vi "ramped_pulse.vi"(8 "error in":errorcluster, 10 "d ramp":u16=1, 11 "d stim":u16=1000) -> (0 "error out":errorcluster, 3 "output":dbl[](array[numeric]))   [LabVIEW 2016]
uses:
  <vilib>/Analysis/1siggen.llb/Ramp Pattern by Samples.vi
  <vilib>/Analysis/NI_AALBase.lvlib
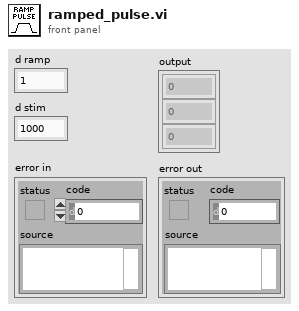
[diagram p1: front panel]
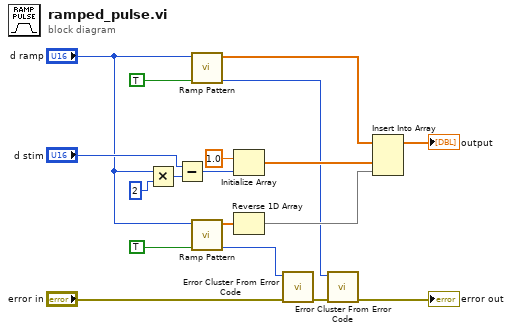
[diagram p0: block diagram]
diagram:
  n1 = Multiply(x="d ramp", y=2 ("d ramp")) -> (x*y=w9:i32)
  n2 = Subtract(x="d stim", y=w9) -> (x-y=w11:i32)
  n3 = call-poly <vilib>:"Ramp Pattern.vi"("exclude end?"=TRUE, "samples"="d ramp") -> ("error"=w4:i32, "Ramp Pattern"=w17:dbl[])  [unwired: 8 in]
  n4 = call-poly <vilib>:"Ramp Pattern.vi"("exclude end?"=TRUE, "samples"="d ramp") -> ("error"=w13:i32, "Ramp Pattern"=w15:dbl[])  [unwired: 8 in]
  n5 = Initialize Array(1.0 ("element"), w11) -> (w16:dbl[])
  n6 = Reverse 1D Array(array=w15) -> (reversed array=w14:dbl[])
  n7 = call <vilib>:"Error Cluster From Error Code.vi"("error in (no error)"="error in", "error code (0)"=w13) -> ("error out"=w6:errorcluster)  [unwired: 7 in]
  n8 = call <vilib>:"Error Cluster From Error Code.vi"("error in (no error)"=w6, "error code (0)"=w4) -> ("error out"=→"error out":errorcluster)  [unwired: 7 in]
  n9 = Insert Into Array(array=w17, new element #1=w16, new element #2=w14) -> (→"output":dbl[])  [unwired: 1 in]
